vi "Read Last Object.vi"(8 "error in":errorcluster, 11 "Buffer in":refnum<data-value>) -> (0 "error out":errorcluster, 1 "found":bool, 2 "element":refnum<class>, 3 "Buffer":refnum<data-value>)   [LabVIEW 2013, in "ObjectBuffer.lvclass"]
doc: "This VI returns data from the ring buffer starting from the oldest data and ending with the newest.\n\nThe data is duplicated at the output so this VI allocates new place in the memory for the output."
uses:
  ObjectBuffer.lvclass
  ObjectBuffer.lvclass/ObjectBuffer.ctl
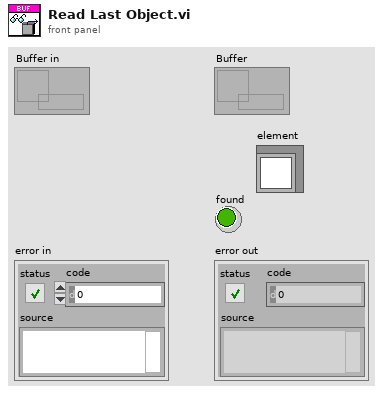
[diagram p1: front panel]
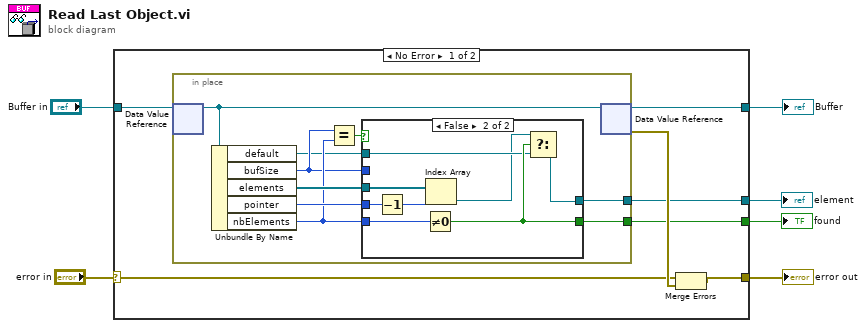
[diagram p0: block diagram]
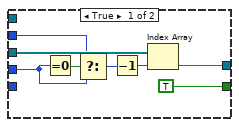
[diagram p2: hidden frame]
diagram:
  n1 = case shown="No Error" "error in" {
    selector: "error in" -> [w8 w39]
    tunnel: "Buffer in" -> [w13 w40]
    tunnel: [w12 w40] -> w5
    tunnel: [w10 w39] -> w2
    tunnel: [w9 _] -> w4
    tunnel: [w7 _] -> w1
    frame No Error {
      n2 = in-place {
        in-place-border: [w20] -> w9
        in-place-border: [w19] -> w7
        n3 = in-place-dvr #1(w13) -> (w22:refnum<class "ObjectBuffer.lvclass">)  [unwired: 1 out]
        n4 = Unbundle By Name(w22) -> ("default"=w14:refnum<class>, "bufSize"=w15:i32, "elements"=w21:refnum<class>[], "pointer"=w18:i32, "nbElements"=w16:i32)
        n5 = Equal?(x=w15, y=w16) -> (x = y?=w17:bool)
        n6 = case shown="False" w17 {
          tunnel: w21 -> [w30 w38]
          tunnel: [w29 w31] -> w20
          tunnel: [TRUE w34] -> w19
          tunnel: w18 -> [w25 w37]
          tunnel: w16 -> [_ w36]
          tunnel: w15 -> [w26 _]
          tunnel: w14 -> [_ w33]
          frame True {
            n7 = Equal To 0?(x=w25) -> (x = 0?=w27:bool)
            n8 = Select(t=w26, s=w27, f=w25) -> (s? t:f=w24:i32)
            n9 = Decrement(x=w24) -> (x-1=w28:i32)
            n10 = Index Array(array=w30, index=w28) -> (element=w29:refnum<class>)
          }
          frame False {
            n11 = Decrement(x=w37) -> (x-1=w35:i32)
            n12 = Not Equal To 0?(x=w36) -> (x != 0?=w34:bool)
            n13 = Index Array(array=w38, index=w35) -> (element=w32:refnum<class>)
            n14 = Select(t=w32, s=w34, f=w33) -> (s? t:f=w31:refnum<class>)
          }
        }
        n15 = in-place-dvr #1(w22) -> (w12:refnum<data-value>, w11:errorcluster)
      }
      n16 = Merge Errors(w8, w11) -> (w10:errorcluster)
    }
    frame Error {
    }
  }
  "error out" <- w2
  "Buffer" <- w5
  "element" <- w4
  "found" <- w1
